vi "Test Call Global Setup only Once.vi"(8 "error in (no error)":errorcluster, 11 "Test Case In":refnum<class "Global Fixture Test.lvclass">) -> (0 "error out":errorcluster, 3 "Test Case Out":refnum<class "Global Fixture Test.lvclass">)   [LabVIEW 2020, in "Global Fixture Test.lvclass"]
uses:
  Global Fixture Test.lvclass
  C:/Program Files (x86)/National Instruments/LabVIEW 2020/vi.lib/Astemes/LUnit/Test Case.lvclass
  Global Fixture Test Double/Global Fixture Test Double.lvclass
  <vilib>/Astemes/LUnit/Test Case.lvclass/Test Case.ctl
  e03a561d-6ba3-4625-bd84-afcdd73d624e.vi
  <vilib>/Astemes/LUnit/Append Pass Result.vi
  <vilib>/Astemes/LUnit/Append Fail Result.vi
  <vilib>/Astemes/LUnit/Describe Comparison.vi
  <vilib>/Astemes/LUnit/Compare Variants.vi
  <vilib>/Astemes/LUnit/Run In UI.vi
  <vilib>/Utility/error.llb/Clear Errors.vi
  <vilib>/Astemes/LUnit/Describe Variant.vi
  <vilib>/Astemes/LUnit/Test Suite.lvclass
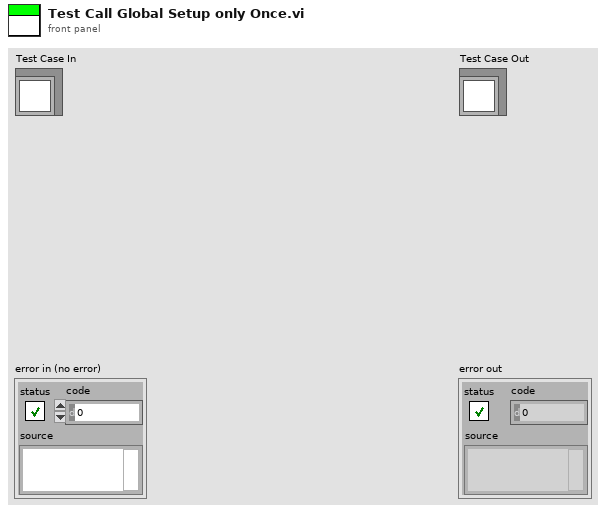
[diagram p1: front panel]
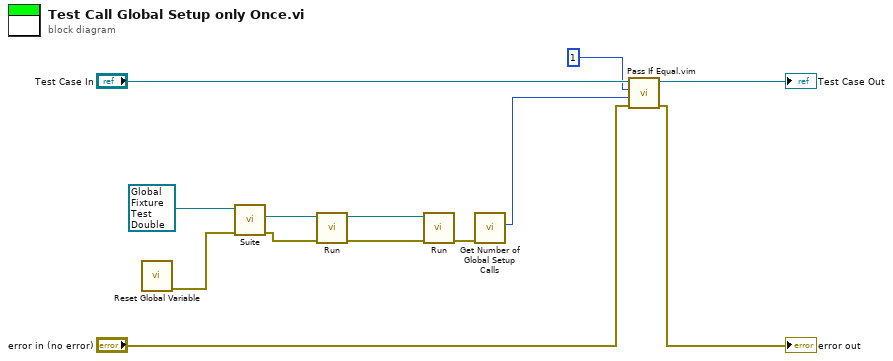
[diagram p0: block diagram]
diagram:
  n1 = call "Reset Global Variable.vi"() -> ("error out"=w8:errorcluster)  [unwired: 11 in]
  n2 = call-dynamic "Suite.vi"("error in (no error)"=w8, "Global Fixture Test Case In"=refnum<class "Global Fixture Test Double.lvclass"> refnum ("Global Fixture Test Double.lvclass")) -> ("error out"=w7:errorcluster, "LUnit Test Suite Out"=w9:refnum<class "Test Suite.lvclass">)  [unwired: 7 in, 1 out]
  n3 = call-dynamic "Run.vi"("error in (no error)"=w7, "LUnit Test Suite In"=w9) -> ("error out"=w3:errorcluster, "LUnit Test Suite In 2"=w4:refnum<class "Test Suite.lvclass">)  [unwired: 6 in, 2 out]
  n4 = call-dynamic "Run.vi"("error in (no error)"=w3, "LUnit Test Suite In"=w4) -> ("error out"=w5:errorcluster)  [unwired: 6 in, 3 out]
  n5 = call "Get Number of Global Setup Calls.vi"("error in (no error)"=w5) -> ("Calls to Setup"=w2:i32)  [unwired: 9 in, 1 out]
  n6 = call "Pass If Equal.vim"("error in (no error)"="error in (no error)", "Actual"=w2, "Expected"=1 ("Calls to Setup"), "LUnit Test Case In"="Test Case In") -> ("error out"=→"error out":errorcluster, "LUnit Test Case Out"=→"Test Case Out":refnum<class "Global Fixture Test.lvclass">)  [unwired: 6 in]
